vi "oa_Extract XY Signal Segment (1 Channel).vi"(0 "XY signal in":cluster{"time/rev/rpm":dbl[], "magnitude":dbl[]}, 1 "X axis selection":u16(ring)=2 items=["Time", "Revolution", "RPM"], 2 "reset? (F)":bool, 5 "trigger indices":T1, 7 "position info in":T2, 11 "error in (no error)":errorcluster, 12 "indices end?":bool) -> (4 "XY signal out":cluster{"time/rev/rpm":dbl[], "magnitude":dbl[]}, 8 "position info out":T2, 14 "reached end?":bool, 15 "error out":errorcluster)   [LabVIEW 2017, in "SoundVib_OAUtility.lvlib"]
uses:
  <vilib>/addons/Sound and Vibration/Order Analysis/Utility/SoundVib_OAUtility.lvlib
  <vilib>/addons/Sound and Vibration/Order Analysis/Misc/OAT Position Info.ctl
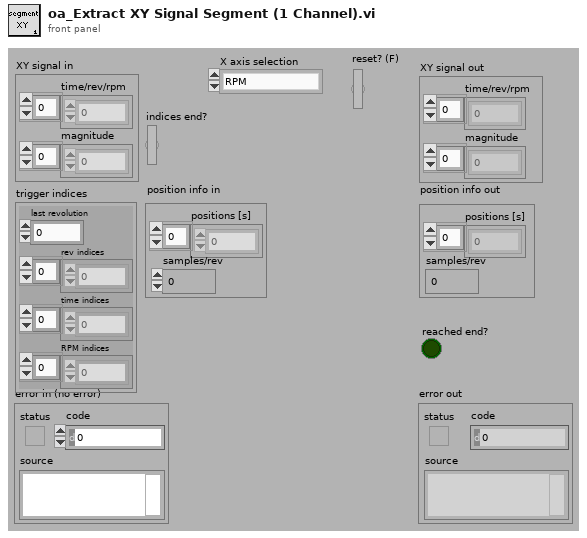
[diagram p1: front panel]
types:
  T1 = cluster{"last revolution":dbl, "rev indices":dbl[], "time indices":dbl[], "RPM indices":dbl[]}
  T2 = typedef "OAT Position Info.ctl" = cluster{"positions [s]":dbl[], "samples/rev":dbl}
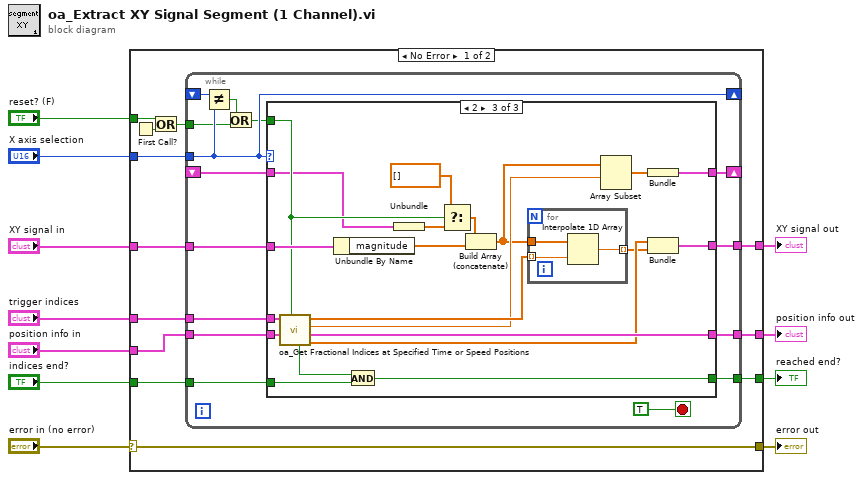
[diagram p0: block diagram]
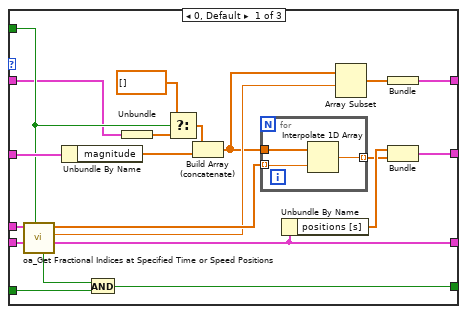
[diagram p2: hidden frame]
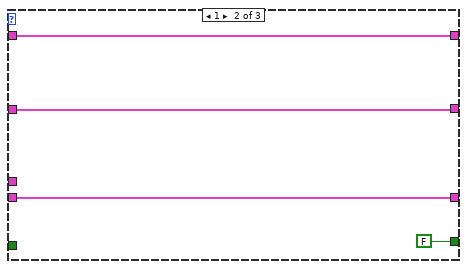
[diagram p3: hidden frame]
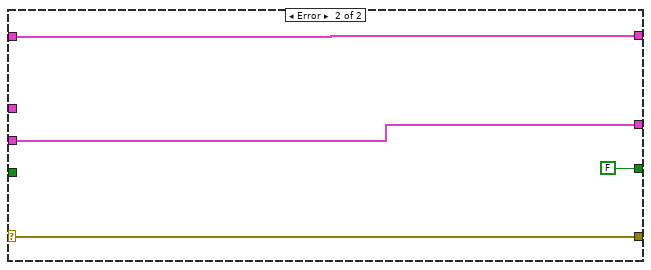
[diagram p4: hidden frame]
diagram:
  n1 = case shown="No Error" "error in (no error)" {
    selector: "error in (no error)" -> [w14 w94]
    tunnel: [w14 w94] -> w10
    tunnel: "reset? (F)" -> [w23 _]
    tunnel: "XY signal in" -> [w19 w93]
    tunnel: [w20 w93] -> w7
    tunnel: "position info in" -> [w16 w92]
    tunnel: "trigger indices" -> [w17 _]
    tunnel: "X axis selection" -> [w21 _]
    tunnel: [w15 w92] -> w3
    tunnel: "indices end?" -> [w13 _]
    tunnel: [w12 FALSE] -> w1
    frame No Error {
      n2 = First Call?() -> (First Call?: T/F=w22:bool)
      n3 = Or(x=w23, y=w22) -> (x .or. y?=w18:bool)
      n4 = while {
        tunnel: w21 -> [w29]
        tunnel: [w38] -> w20
        tunnel: w19 -> [w37]
        tunnel: w18 -> [w27]
        tunnel: w17 -> [w36]
        tunnel: w16 -> [w35]
        tunnel: [w34] -> w15
        shift-right: [w32] -> _
        shift-left: _ -> [w31]
        shift-right: [w29] -> _
        shift-left: _ -> [w30]
        tunnel: w13 -> [w25]
        tunnel: [w24] -> w12
        stop <- TRUE stop-if-true
        n5 = Not Equal?(x=w30, y=w29) -> (x != y?=w26:bool)
        n6 = Or(x=w26, y=w27) -> (x .or. y?=w28:bool)
        n7 = case shown="2" w29 {
          tunnel: [w53 w66 w82] -> w38
          tunnel: w37 -> [w57 w66 w85]
          tunnel: w28 -> [w50 _ w84]
          tunnel: w36 -> [w59 _ w81]
          tunnel: w35 -> [w58 w65 w80]
          tunnel: [w55 w65 w79] -> w34
          tunnel: [w51 w64 w83] -> w32
          tunnel: w31 -> [w42 w64 w70]
          tunnel: w25 -> [w41 _ w69]
          tunnel: [w39 FALSE w67] -> w24
          frame 0, Default {
            n8 = call <vilib>:"oa_Get Fractional Indices at Specified Time or Speed Positions.vi"("reset? (F)"=w50, "position info in"=w58, "trigger indices"=w59) -> ("position info out"=w55:T2, "buffer index"=w52:dbl, "fractional indices out"=w56:dbl[], "indices buffer empty?"=w40:bool)  [unwired: 4 in, 1 out]
            n9 = Unbundle By Name(w57) -> ("magnitude"=w45:dbl[])
            n10 = And(x=w40, y=w41) -> (x .and. y?=w39:bool)
            n11 = Unbundle(w42) -> (w47:dbl[])
            n12 = Select(t=dbl[] [], s=w50, f=w47) -> (s? t:f=w46:dbl[])
            n13 = Build Array (concatenate)(w46, w45) -> (w44:dbl[])
            n14 = for {
              tunnel: w44 -> [w62]
              tunnel: w56 -> [w61] mode=indexing
              tunnel: [w60] -> w49 mode=indexing
              n15 = Interpolate 1D Array(1:w61, 2:w62) -> (0:w60:dbl)
            }
            n16 = Unbundle By Name(w55) -> ("positions [s]"=w54:dbl[])
            n17 = Array Subset(array=w44, index=w52) -> (w48:dbl[])  [unwired: 1 in]
            n18 = Bundle(w48) -> (w51:cluster{dbl[]})  [unwired: 1 in]
            n19 = Bundle("positions [s]"=w54, w49) -> (w53:cluster{"positions [s]":dbl[], dbl[]})  [unwired: 1 in]
          }
          frame 1 {
          }
          frame 2 {
            n20 = call <vilib>:"oa_Get Fractional Indices at Specified Time or Speed Positions.vi"("reset? (F)"=w84, "position info in"=w80, "trigger indices"=w81) -> ("rpm indices"=w78:dbl[], "position info out"=w79:T2, "buffer index"=w86:dbl, "fractional indices out"=w87:dbl[], "indices buffer empty?"=w68:bool)  [unwired: 4 in]
            n21 = Unbundle By Name(w85) -> ("magnitude"=w72:dbl[])
            n22 = And(x=w68, y=w69) -> (x .and. y?=w67:bool)
            n23 = Unbundle(w70) -> (w75:dbl[])
            n24 = Select(t=dbl[] [], s=w84, f=w75) -> (s? t:f=w73:dbl[])
            n25 = Build Array (concatenate)(w73, w72) -> (w71:dbl[])
            n26 = for {
              tunnel: w71 -> [w90]
              tunnel: w87 -> [w89] mode=indexing
              tunnel: [w88] -> w77 mode=indexing
              n27 = Interpolate 1D Array(1:w89, 2:w90) -> (0:w88:dbl)
            }
            n28 = Array Subset(array=w71, index=w86) -> (w76:dbl[])  [unwired: 1 in]
            n29 = Bundle(w76) -> (w83:cluster{dbl[]})  [unwired: 1 in]
            n30 = Bundle("rpm indices"=w78, w77) -> (w82:cluster{"rpm indices":dbl[], dbl[]})  [unwired: 1 in]
          }
        }
      }
    }
    frame Error {
    }
  }
  "error out" <- w10
  "XY signal out" <- w7
  "position info out" <- w3
  "reached end?" <- w1
